vi "Queue Comms Flush Enqueue.vi"(8 "error in (no error)":errorcluster, 11 "element":T1) -> (0 "error out":errorcluster)   [LabVIEW 2014, in "Testing UI 1.lvlib"]
doc: "This subVI flushes the queue then enqueues an element in to the communications queue to be handleds"
uses:
  Testing UI 1.lvlib
  Private Controls/Module Data.ctl
  Private Controls/Module Action.ctl
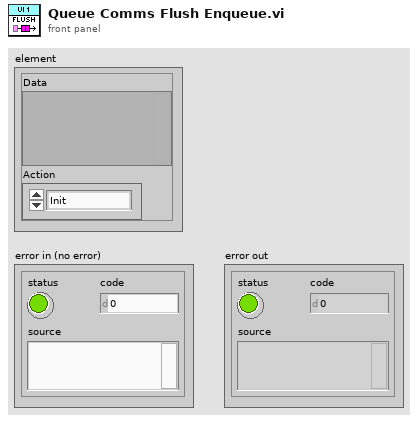
[diagram p1: front panel]
types:
  T1 = typedef "Testing UI 1.lvlib/Module Data.ctl" = cluster{"Data":variant, "Action":T2}
  T2 = typedef "Testing UI 1.lvlib/Module Action.ctl" = enum8{"Init", "Error", "Exit", "HideShow FP", "Send Control Vals", "New Message Line", "Update System Log", "Load APU Setup Data", "Update APU Name", "Set Testing Type", "Threshold ALERT", "Set Rapid OpenORClose", "Engine Start Val Change", "Fault Trip Run Updater", " ---------------UI 4 APIs ---------------", "UI 4 Engine Start Val Change", "UI 4 Fuel Pressure Reg Val Change", "U1 4 APU & ECU Control Val Change", "UI 4 Bleed Load Val Change", "UI4 Testing Controls Val Change", "UI4 Break Out Val Change", "UI4 Crash Log Val Change", "UI4 Log Data Val Change", "UI4 Sampes-Sec Val Change", "Update Run Count", "Config Interactive Ctrls"}
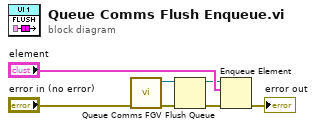
[diagram p0: block diagram]
diagram:
  n1 = call "Queue Comms FGV.vi"("error in (no error)"="error in (no error)") -> ("error out"=w4:errorcluster, "Queue out"=w3:refnum<queue>)  [unwired: 9 in]
  n2 = Flush Queue(queue=w3, error in (no error)=w4) -> (queue out=w2:refnum<queue>, error out=w1:errorcluster)  [unwired: 1 out]
  n3 = Enqueue Element(queue=w2, element="element", error in (no error)=w1) -> (error out=→"error out":errorcluster)  [unwired: 1 in, 2 out]
